vi "Untitled 1.vi"() -> ()   [LabVIEW 2021]
uses:
  Mete.ctl
  Odo Velocity.ctl
  R.ctl
  P.ctl
  N.ctl
  D.ctl
  Gas.ctl
panel:
  out "Waveform Chart":dbl(graph)
  in  "Boolean 5":bool
  in  "Thermometer":T1
  out "Boolean 4":T2
  out "Boolean 3":T3
  out "Boolean 2":T4
  out "Boolean":T5
  out "Km/h":T6 scale=0.0..250.0
  out "Gauge":T7 scale=0.0..650.0
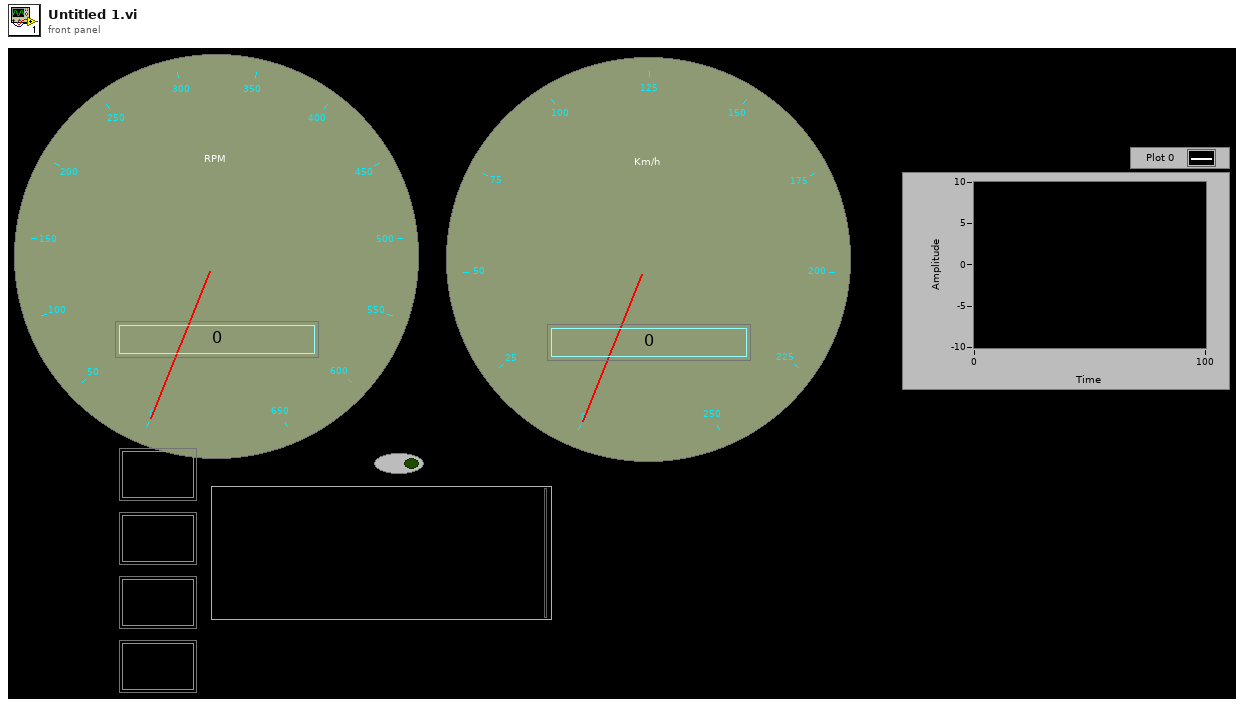
[diagram p1: front panel]
types:
  T1 = typedef "Gas.ctl" = dbl
  T2 = typedef "D.ctl" = bool
  T3 = typedef "N.ctl" = bool
  T4 = typedef "P.ctl" = bool
  T5 = typedef "R.ctl" = bool
  T6 = typedef "Odo Velocity.ctl" = u16
  T7 = typedef "Mete.ctl" = u16
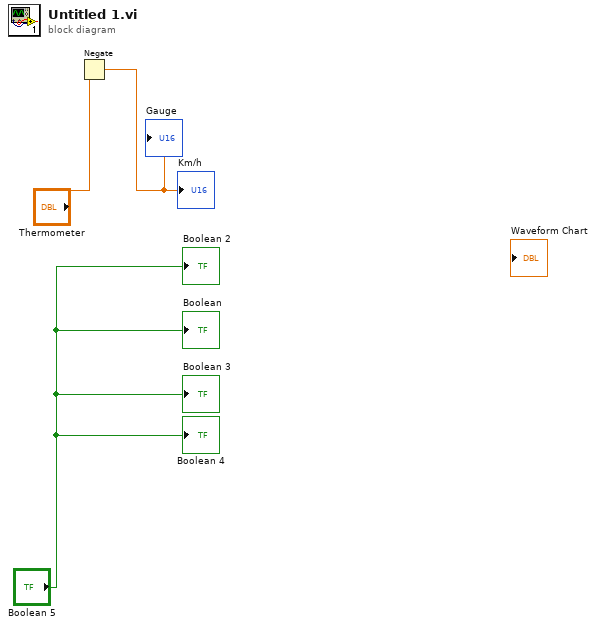
[diagram p0: block diagram]
diagram:
  n1 = Negate(x="Thermometer") -> (-x=→"Gauge" →"Km/h":T1)
  "Boolean" <- "Boolean 5"
  "Boolean 2" <- "Boolean 5"
  "Boolean 3" <- "Boolean 5"
  "Boolean 4" <- "Boolean 5"
